vi "Hessian.vi"() -> ()   [LabVIEW 2016]
uses:
  <vilib>/Analysis/baseanly.llb/Matrix Type of Inverse Matrix.ctl
  <vilib>/Analysis/7linalg.llb/Real Eigenvalues and Vectors.vi
  <vilib>/Analysis/baseanly.llb/Real Inverse Matrix.vi
  <vilib>/Analysis/NI_AALBase.lvlib
  <vilib>/Analysis/NI_AALPro.lvlib
panel:
  out "1/evals 2":dbl[](array[numeric])=[1.4932539206430082e-06, 1.382955062497276e-06, 3.31245858032921e-05, 4.541745455416717e-05, 0.002247934818473577, 0.08229727726463083, 0.00011474803820043863, 0.00010265593626842863] min=0.0 max=127.0 format="%#_3e"
  out "Sigma^2":dbl=1.6900000000000002
  out "Eigenvectors":dbl[][](array[numeric])=[[-0.00020649614341403647, 1.804999423511327e-05, -0.00916385577476654, 0.0013766013238125888, 0.9941522795930202, 0.10997992901820673, -0.013406740927156532, 0.01032398476258208], [0.19772846971866231, -0.8926223197896882, 0.17960258283952701, -0.02058981753908376, 0.023024168785321354, 0.02516608965099213, 0.024100143633845477, -0.0007190045606287962], [-1.4840425152786332e-05, 7.893534255554087e-05, -0.0037370398104449084, 8.808546408354794e-05, -0.0055141562347290896, 0.9876192228475299, 0.002580998218309943, -0.0021147545531178496], [0.0014851878980094934, -0.0016248578442849774, 0.9045641317250716, -0.008327106118336201, 0.0011512099110235958, 0.0004206684875452048, -0.02079076752113622, 0.02663852705622989], [0.000581766684012567, 0.002969657177653981, -0.3113277704772086, 0.06374282319656148, 0.09021079692024259, 0.09278730422790732, 0.7669104181831797, -0.853031578001316], [-0.0017864996443897603, -0.0009704499245489904, -0.16077024910167798, 0.025614336862171058, 0.050280749799090564, 0.05247930198687596, 0.6403547168597442, 0.5210672975999243], [-0.006533548485729128, 0.007763918404825544, -0.025829200624953648, -0.9972521474393052, 0.0016906290087462263, 0.0018061357652201019, 0.007824616026657459, 0.0013663258900481177], [0.9802321083954854, -0.45072464812551094, -0.16115055334432934, 0.016544745174367253, -0.02074612061849958, -0.022635232615964136, -0.023098642172903302, 0.0017165426231599626]] format="%_4g"
  in  "Sigma":dbl=1.3 format="%g"
  out "1/evals":dbl[](array[numeric])=[8.835822015639101e-07, 8.18316605027974e-07, 1.9600346629166924e-05, 2.687423346400424e-05, 0.0013301389458423532, 0.04869661376605374, 6.789824745588084e-05, 6.07431575552832e-05] min=0.0 max=127.0 format="%#_3e"
  out "Eigenvalues":dbl[](array[numeric])=[1131756.6132840095, 1222020.9071350999, 51019.505875060284, 37210.363649605686, 751.8011581615016, 20.535308775352608, 14727.920638154666, 16462.75959707702] min=0.0 max=127.0
  out "message":string="No Error"
  out "error":i32
  in  "Fn":u16(ring) items=["Error", "Test"]
  out "Intensity Graph":dbl[][](graph)=[[0.0013588328784681707, 3.296041280378604e-07, 0.0052709371261644945, 3.723858404677595e-05, 4.6556876395672e-06, 1.3844006787932266e-06, 2.3238776839930144e-06, 2.582079275282164e-07], [3.775893787105628e-05, 9.023661451008171e-07, 0.0012367631798337764, 8.73651785168589e-06, -1.8117432616783578e-06, 7.746604228709897e-07, 5.289955267067581e-07, 1.5665509921069012e-08], [0.0002756727254175688, 3.677577761782894e-06, 0.048679556757268753, 0.00015285512304405243, -0.0001302907736563917, -2.9232928682661124e-05, -5.756365362611478e-06, -1.9268713756308398e-07], [1.7554409758497363e-06, -2.5475248993647896e-08, 2.0665446370645266e-05, 1.9239368175681962e-05, -1.3394412300990445e-06, -2.1808527616860838e-08, -1.8003426969493122e-08, -2.1354920037894622e-08], [0.00014089735245484958, 5.784531799872248e-07, 0.0045541618169812025, 3.237553513873929e-05, 5.373440810695152e-05, 2.557981842519164e-06, 2.095712277358176e-06, -7.984286091050768e-08], [7.861313424956107e-05, 5.538385437395726e-08, 0.0025757600440660367, 1.8197693303859542e-05, -3.1612999442316723e-06, 6.353087575423601e-05, 9.246980321958817e-07, 1.390291028533225e-07], [2.697164862806379e-06, 1.6114477088158595e-07, 8.869450559227879e-05, 6.274545800398178e-07, -5.058852404397753e-08, 2.801719082383122e-07, 2.688354782149025e-05, 1.4229325274942336e-07], [-3.3998610317428576e-05, -1.189689615513505e-07, -0.0011123689134883747, -7.863217709798505e-06, 1.5344817675588926e-06, -7.287350544201174e-07, -4.287867760235751e-07, 8.903940601483454e-07]]
  out "Hinv":dbl[][](array[numeric])=[[0.0013588328784681707, 3.296041280378604e-07, 0.0052709371261644945, 3.723858404677595e-05, 4.6556876395672e-06, 1.3844006787932266e-06, 2.3238776839930144e-06, 2.582079275282164e-07], [3.775893787105628e-05, 9.023661451008171e-07, 0.0012367631798337764, 8.73651785168589e-06, -1.8117432616783578e-06, 7.746604228709897e-07, 5.289955267067581e-07, 1.5665509921069012e-08], [0.0002756727254175688, 3.677577761782894e-06, 0.048679556757268753, 0.00015285512304405243, -0.0001302907736563917, -2.9232928682661124e-05, -5.756365362611478e-06, -1.9268713756308398e-07], [1.7554409758497363e-06, -2.5475248993647896e-08, 2.0665446370645266e-05, 1.9239368175681962e-05, -1.3394412300990445e-06, -2.1808527616860838e-08, -1.8003426969493122e-08, -2.1354920037894622e-08], [0.00014089735245484958, 5.784531799872248e-07, 0.0045541618169812025, 3.237553513873929e-05, 5.373440810695152e-05, 2.557981842519164e-06, 2.095712277358176e-06, -7.984286091050768e-08], [7.861313424956107e-05, 5.538385437395726e-08, 0.0025757600440660367, 1.8197693303859542e-05, -3.1612999442316723e-06, 6.353087575423601e-05, 9.246980321958817e-07, 1.390291028533225e-07], [2.697164862806379e-06, 1.6114477088158595e-07, 8.869450559227879e-05, 6.274545800398178e-07, -5.058852404397753e-08, 2.801719082383122e-07, 2.688354782149025e-05, 1.4229325274942336e-07], [-3.3998610317428576e-05, -1.189689615513505e-07, -0.0011123689134883747, -7.863217709798505e-06, 1.5344817675588926e-06, -7.287350544201174e-07, -4.287867760235751e-07, 8.903940601483454e-07]] format="%_4g"
  out "Hessian":dbl[][](array[numeric])=[[768.1092494031816, 105.9674201719929, -66.95762615560596, -667.5771851671896, -237.1217514429702, -42.19489133028276, -67.46137102009442, -259.0052375044394], [-25229.312402526462, 1232361.413315619, -25236.89541052221, -252210.73887367494, -24680.01693193145, -25302.02746573096, -25167.95691875373, -20116.37555109225], [-5.360080282734714, -110.3167935028182, 19.81885315771592, -172.1330995252401, 40.883386184020765, 8.923198941523935, 3.3544680597685783, 5.3925309808633415], [-155.9047645116607, 1456.4126780847173, -105.04993399607086, 51312.416882431935, 1044.378142722735, -71.47246090077886, -60.86289191742366, 1342.0512450856845], [-1129.2991123177387, -4833.340458050728, -1104.2101645157843, -11212.126494726248, 15479.512892216719, -1027.5168166860028, -1196.3565654493636, 1644.3577448601588], [-764.7092905429531, 2605.9244554197394, -765.4892946922232, -7650.955094362643, -915.5238396179044, 15380.869692396716, -652.5979013805028, -2552.6685208809854], [-0.31926522492398135, -7372.0645248052115, -0.5587223981251555, -8.391731203261088, -57.33032085863954, -138.99118559912438, 37259.044758319425, -5808.306432026456], [19205.34341927116, 50662.151069492014, 19179.46766127887, 191969.98709744227, 20492.97977223219, 19816.898979215126, 17185.010538693037, 1121389.2210023976]] format="%_4g"
  in  "d":dbl=0.001 format="%_4g"
  in  "d rel":dbl[](array[numeric])=[1.0, 1.0, 1.0, 0.1, 1.0, 1.0, 1.0, 1.0] format="%_4g"
  in  "Array In":dbl[](array[numeric])=[7.044400000000002, 0.4286399999999992, 0.536279999999991, 1.5500139999999916, 0.17059000000000035, 0.35147, 0.30979, 0.04216999999999992] format="%_6g"
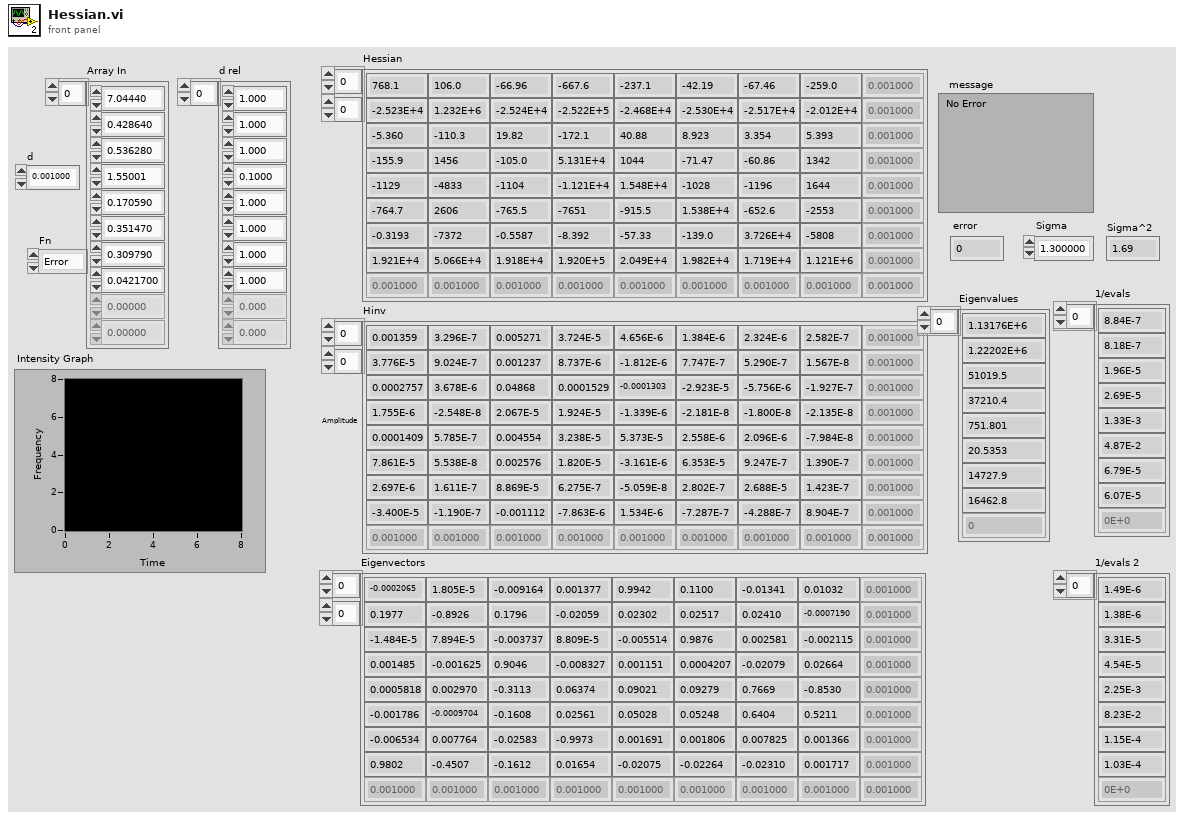
[diagram p1: front panel]
types:
  T1 = typedef "NI_AALBase.lvlib/Matrix Type of Inverse Matrix.ctl" = enum32{"General", "Positive Definite", "Lower Triangular", "Upper Triangular"}
  T2 = typedef "NI_Matrix.lvlib/ComplexMatrix.ctl" = cdb[][]
  T3 = typedef "NI_Matrix.lvlib/RealMatrix.ctl" = dbl[][]
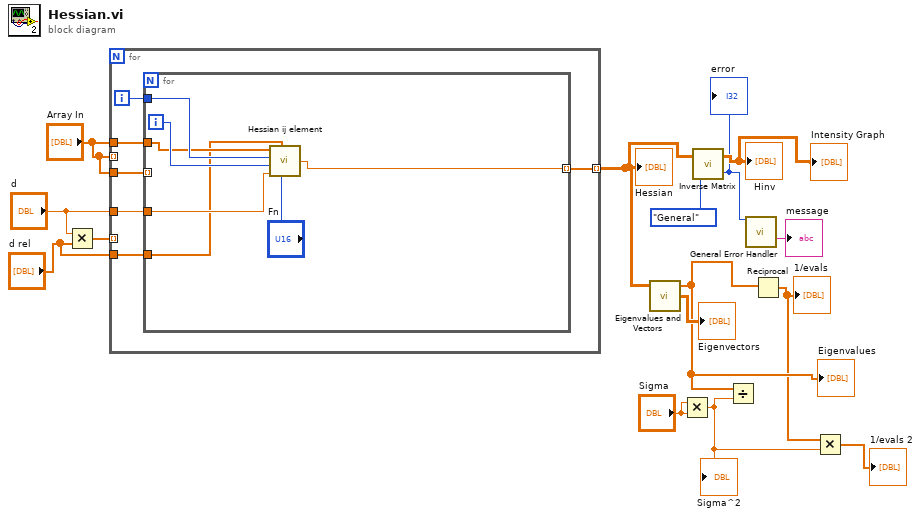
[diagram p0: block diagram]
diagram:
  n1 = Multiply(x="d", y="d rel") -> (x*y=w15:dbl[])
  n2 = for {
    tunnel: "Array In" -> [w21]
    tunnel: w15 -> [_] mode=indexing
    tunnel: "d" -> [w19]
    tunnel: "d rel" -> [w18]
    tunnel: [w17] -> w7 mode=indexing
    tunnel: "Array In" -> [_] mode=indexing
    tunnel: "Array In" -> [w16]
    i -> [w20]
    n3 = for {
      tunnel: w21 -> [w25]
      tunnel: w20 -> [w28]
      tunnel: w19 -> [w26]
      tunnel: w18 -> [w24]
      tunnel: [w22] -> w17 mode=indexing
      tunnel: w16 -> [_] mode=indexing
      i -> [w27]
      n4 = call "Hessian ij element.vi"("Fn"="Fn", "d rel"=w24, "d"=w26, "j"=w27, "i"=w28, "Array"=w25) -> ("Hij"=w22:dbl)
    }
  }
  "Hessian" <- w7
  n5 = call-poly <vilib>:"Eigenvalues and Vectors.vi"("Input Matrix"=w7) -> ("Eigenvectors"=→"Eigenvectors":T2, "Eigenvalues"=w3:cdb[])  [unwired: 2 in, 1 out]
  "Eigenvalues" <- w3
  n6 = Multiply(x="Sigma", y="Sigma") -> (x*y=w2:dbl)
  "Sigma^2" <- w2
  n7 = call-poly <vilib>:"Inverse Matrix.vi"("matrix type"=Matrix_Type_of_Inverse_Matrix."General", "Input Matrix"=w7) -> ("error"=w9:i32, "Inverse Matrix"=→"Hinv" →"Intensity Graph":T3)
  "error" <- w9
  n8 = Divide(x=w3, y=w2) -> ()  [unwired: 1 out]
  n9 = call <vilib>:"General Error Handler.vi"("[error code] (0)"=w9) -> ("message"=→"message":string)  [unwired: 10 in, 4 out]
  n10 = Reciprocal(x=w3) -> (1/x=w1:cdb[])
  "1/evals" <- w1
  n11 = Multiply(x=w1, y=w2) -> (x*y=→"1/evals 2":cdb[])
